vi "csv-log-data.vi"(0 "log file Byte Stream File in":refnum<file>, 1 "log file path":path, 5 "Data Array In":dbl[](array[numeric]), 9 "File Open?":bool=TRUE, 11 "error in (no error)":errorcluster, 12 "Datalogging options":T1={"Include Timestamp"=TRUE, "Include milliseconds"=FALSE, "data-precision"=3}, 13 "Override Format Array?":bool, 14 "Format Array Override":string="%.2f") -> (3 "log file path":path, 4 "log file Byte Stream File out":refnum<file>, 6 "time string":string, 8 "Logged CSV out":string, 15 "error out":errorcluster)   [LabVIEW 2023]
panel:
  out "format array to string":string="%.2f"
  out "datapoints string":string
  # "If \"File Open\" byte stream is used\nelse File Path is used"
  # "Current Timestamp for Logging"
  # "If overriding format array \"Format Array Override\"\nmust have valid format string (%.2f) for float with \n2 digit precision after decimal point"
  # "This is the string that will be logged to file"
  # "The format string used \nto format array data to \ndatapoints string"
  # "The formated string created from Data Array In"
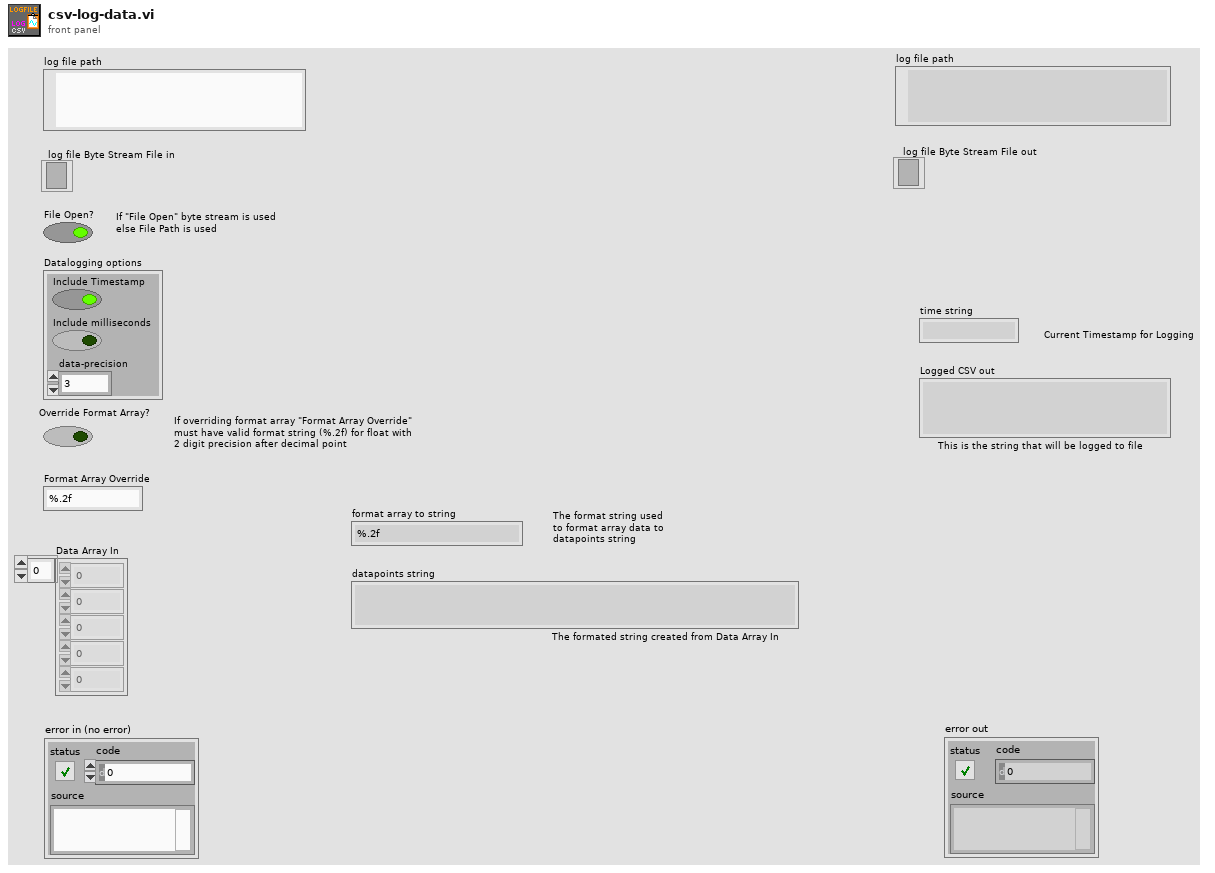
[diagram p1: front panel]
types:
  T1 = cluster{"Include Timestamp":bool, "Include milliseconds":bool, "data-precision":i32}
  T2 = enum16{"open", "replace", "create", "open or create", "replace or create", "replace or create with confirmation"}
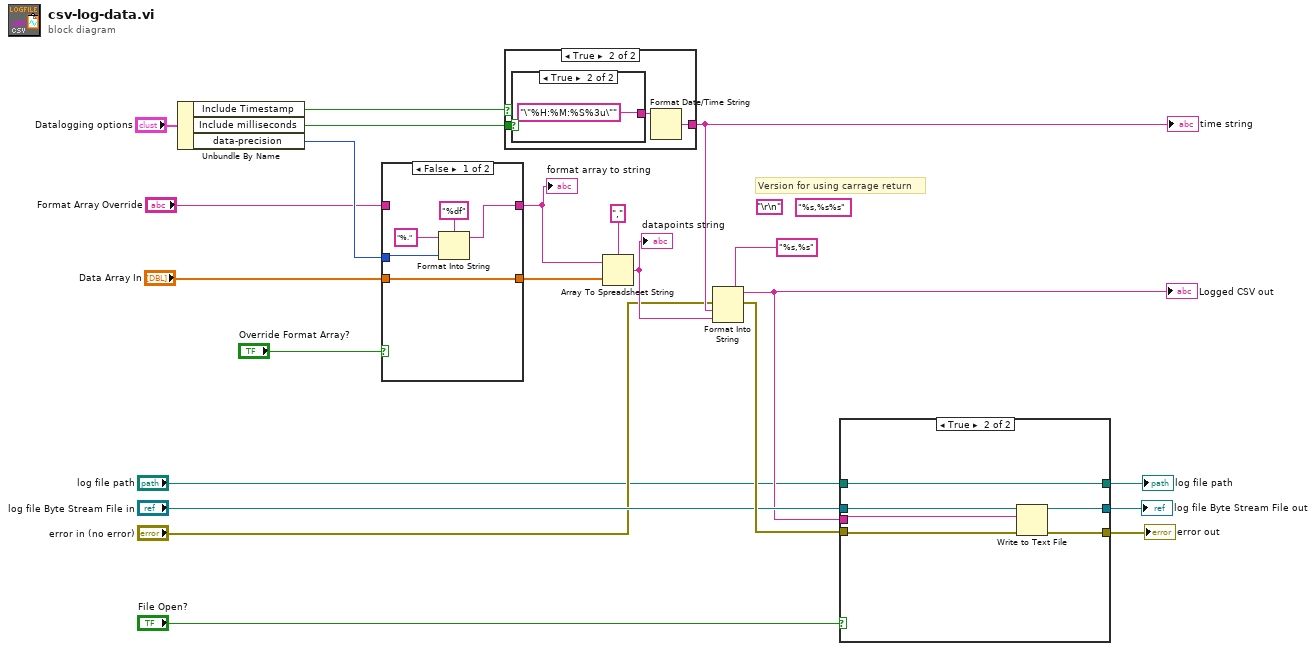
[diagram p0: block diagram]
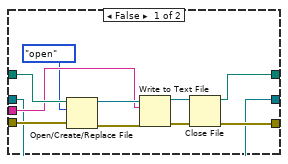
[diagram p3: hidden frame]
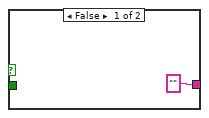
[diagram p4: hidden frame]
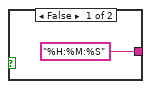
[diagram p5: hidden frame]
diagram:
  (unwired) "%s,%s%s" ("format string")
  (unwired) "\r\n"
  # "Version for using carrage return"
  n1 = Unbundle By Name("Datalogging options") -> ("Include Timestamp"=w20:bool, "Include milliseconds"=w21:bool, "data-precision"=w22:i32)
  n2 = case shown="False" "Override Format Array?" {
    tunnel: w22 -> [w25 _]
    tunnel: [w24 w29] -> w3
    tunnel: "Format Array Override" -> [_ w29]
    tunnel: "Data Array In" -> [w23 w28]
    tunnel: [w23 w28] -> w1
    frame False {
      n3 = Format Into String(format string="%df", initial string="%.", w25) -> (resulting string=w24:string)  [unwired: 1 in, 1 out]
    }
    frame True {
    }
  }
  "format array to string" <- w3
  n4 = case shown="True" w20 {
    tunnel: ["" ("date/time string") w33] -> w18
    tunnel: w21 -> [_ w31]
    frame False {
    }
    frame True {
      n5 = case shown="True" w31 {
        tunnel: ["%H:%M:%S" ("time format string (%c)") "\"%H:%M:%S%3u\"" ("time format string (%c)")] -> w32
        frame False {
        }
        frame True {
        }
      }
      n6 = Format Date/Time String(time format string (%c)=w32) -> (date/time string=w33:string)  [unwired: 2 in]
    }
  }
  "time string" <- w18
  n7 = Array To Spreadsheet String(delimiter (Tab)=",", array=w1, 3:w3) -> (spreadsheet string=w17:string)
  "datapoints string" <- w17
  n8 = Format Into String "Format Into String"(format string="%s,%s", error in="error in (no error)", w18, w17) -> (resulting string=w11:string, error out=w13:errorcluster)  [unwired: 1 in]
  "Logged CSV out" <- w11
  n9 = case shown="True" "File Open?" {
    tunnel: [w42 w52] -> w15
    tunnel: [w36 w51] -> w14
    tunnel: w13 -> [w38 w50]
    tunnel: "log file Byte Stream File in" -> [w36 w49]
    tunnel: w11 -> [w39 w48]
    tunnel: "log file path" -> [w40 w47]
    tunnel: [w41 w47] -> w7
    frame False {
      n10 = Open/Create/Replace File(file path (use dialog)=w40, error in=w38, operation (0:open)=T2."open") -> (refnum out=w44:refnum<file>, error out=w43:errorcluster)  [unwired: 3 in, 1 out]
      n11 = Write to Text File(file (use dialog)=w44, text=w39, error in=w43) -> (refnum out=w45:refnum<file>, error out=w46:errorcluster)  [unwired: 1 in, 1 out]
      n12 = Close File(refnum=w45, error in=w46) -> (path=w41:path, error out=w42:errorcluster)
    }
    frame True {
      n13 = Write to Text File(file (use dialog)=w49, text=w48, error in=w50) -> (refnum out=w51:refnum<file>, error out=w52:errorcluster)  [unwired: 1 in, 1 out]
    }
  }
  "error out" <- w15
  "log file Byte Stream File out" <- w14
  "log file path" <- w7
